vi "Write FPGA Outputs.vi"(0 "FPGA Ref":T1, 1 "Tank CMDs":T2, 2 "App Config":T3={"Location"="", "Profiles Path"=path "", "Current Profile"="", "CA Number"="", "Controller Type:"=enum."Kuhnke", "Stagger Time (ms)"=0, "Tank 1 Fuel"="", "Tank 2 Fuel"="", "Serial Numbers"={"Position 1 SN"="", "Position 2 SN"="", "Poaition 3 SN"="", "Position 4 SN"="", "Position 5 SN"="", "Position 6 SN"=""}, "Pumps Present"={"Pump 1"=FALSE, "Pump 2"=FALSE, "Pump 3"=FALSE, "Pump 4"=FALSE, "Pump 5"=FALSE, "Pump 6"=FALSE}, "VoltCtrlRef"="", "VoltageSelect"=FALSE, "Watlow Present"=FALSE, "Temp 1"=0, "Temp 2"=0, "Voltage Scale"={"V_FFm"=10.0, "V_FFb"=0.0}, "Pressure Scale"={"Pres_FFm"=0.0, "Pres_FFb"=0.0}, "Temp Tolerance"=0.0, "Target Voltage"=0.0, "Target Pressure"=0.0, "Data Log Init"={"Data Path"=path "", "Data Log Rate (S/s)"=0, "AKLH Rate (Hours/S)"=0.0, "Sync Time Offset (min)"=0, "IP Last 3"=0, "WebDAV IP"=""}, "Email Handler IP"="", "ADC Check"=FALSE, "3 Pump Tank"=FALSE, "Freq Flow?"=FALSE, "Profile Temp Control"=FALSE, "Read Controller Diag"=FALSE, "FFT Min Freq."=0, "FFT Max Freq."=0, "Speed by Current"=FALSE, "Watlow is F4T?"=FALSE, "Test Stop Time"=0.0, "Stop Time Enable"=TRUE, "Timers Include Off-Time"=FALSE, "Pump Timer Email"={"Enable"=FALSE, "Hour to Send"=0}, "Reset Step on Startup"=FALSE}, 3 "Power Relay":T7, 5 "Voltage Enable":bool, 6 "Run Profile":bool) -> (14 "FPGA Ref OUT":T1)   [LabVIEW 2019]
uses:
  Type Defs/App Config.ctl
  Type Defs/Controller Names.ctl
  Data Logger/Data Log Init.ctl
  Type Defs/Pump Timer Email.ctl
  Controls/Tank CMDs.ctl
  Controls/FPGA_Reference.ctl
  <vilib>/Utility/error.llb/Error Cluster From Error Code.vi
  <vilib>/rvi/errors/niLvFpgaAdjustHostInterfaceError.vi
  <vilib>/rvi/interface/nirviReadWriteControl/nirviReadWriteControl.xnode
  FPGA/bitfiles/TI sbRIO PWM (FPGA) v1.0.lvbitx
  NiFpgaLv.dll
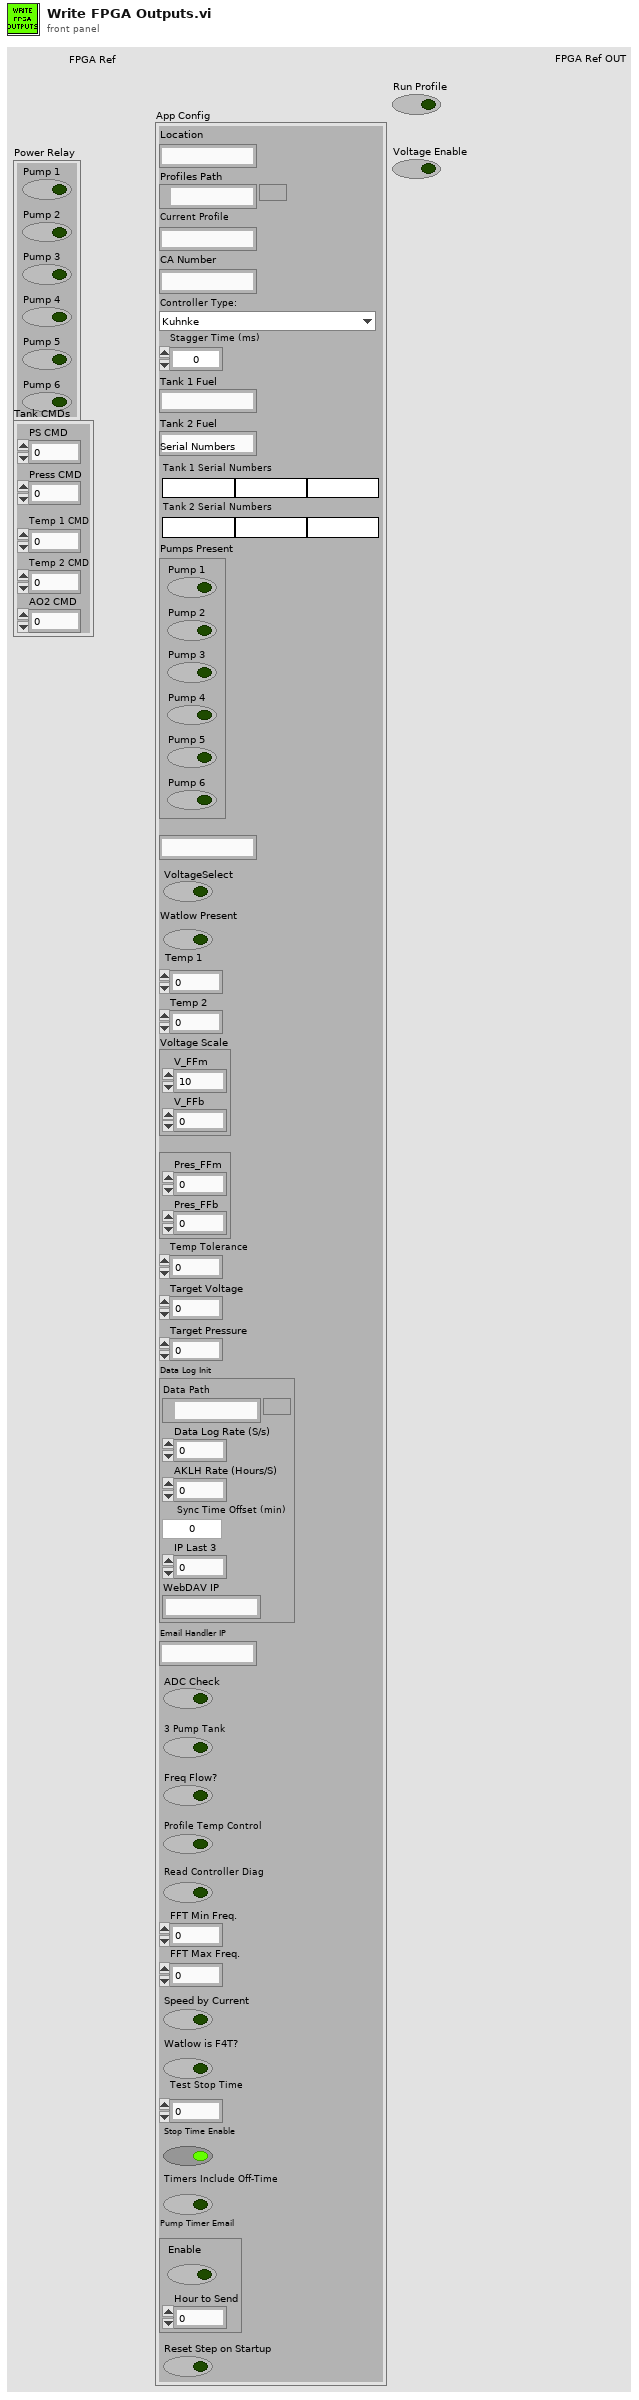
[diagram p1: front panel]
types:
  T1 = typedef "FPGA_Reference.ctl" = refnum<k20>
  T2 = typedef "Tank CMDs.ctl" = cluster{"PS CMD":dbl, "Press CMD":dbl, "Temp 1 CMD":dbl, "Temp 2 CMD":dbl, "AO2 CMD":dbl}
  T3 = typedef "App Config.ctl" = cluster{"Location":string, "Profiles Path":path, "Current Profile":string, "CA Number":string, "Controller Type:":T4, "Stagger Time (ms)":i32, "Tank 1 Fuel":string, "Tank 2 Fuel":string, "Serial Numbers":cluster{"Position 1 SN":string, "Position 2 SN":string, "Poaition 3 SN":string, "Position 4 SN":string, "Position 5 SN":string, "Position 6 SN":string}, "Pumps Present":cluster{"Pump 1":bool, "Pump 2":bool, "Pump 3":bool, "Pump 4":bool, "Pump 5":bool, "Pump 6":bool}, "VoltCtrlRef":string, "VoltageSelect":bool, "Watlow Present":bool, "Temp 1":i16, "Temp 2":i16, "Voltage Scale":cluster{"V_FFm":dbl, "V_FFb":dbl}, "Pressure Scale":cluster{"Pres_FFm":dbl, "Pres_FFb":dbl}, "Temp Tolerance":dbl, "Target Voltage":dbl, "Target Pressure":dbl, "Data Log Init":T5, "Email Handler IP":string, "ADC Check":bool, "3 Pump Tank":bool, "Freq Flow?":bool, "Profile Temp Control":bool, "Read Controller Diag":bool, "FFT Min Freq.":i32, "FFT Max Freq.":i32, "Speed by Current":bool, "Watlow is F4T?":bool, "Test Stop Time":dbl, "Stop Time Enable":bool, "Timers Include Off-Time":bool, "Pump Timer Email":T6, "Reset Step on Startup":bool}
  T4 = typedef "Controller Names.ctl" = enum16{"Kuhnke", "Helbako BLDC", "Conti", "Hella BLDC OL PWM", "Hella BLDC Turbine OL PWM", "Hella BLDC Pressure", "Helbako (old)", "TI PWM", "PSA", "Hella Gas", "Hella Diesel", "8 Comm", "10 Comm", "8 Comm Hella", "10 Comm Hella", "8 Comm Omron", "10 Comm Omron", "8 Comm Nissan", "10 Comm Nissan", "8 Comm Hella (for FCA)", "Mazda BLDC", "CMFB"}
  T5 = typedef "Data Log Init.ctl" = cluster{"Data Path":path, "Data Log Rate (S/s)":u32, "AKLH Rate (Hours/S)":dbl, "Sync Time Offset (min)":i32, "IP Last 3":i32, "WebDAV IP":string}
  T6 = typedef "Pump Timer Email.ctl" = cluster{"Enable":bool, "Hour to Send":u8}
  T7 = cluster{"Pump 1":bool, "Pump 2":bool, "Pump 3":bool, "Pump 4":bool, "Pump 5":bool, "Pump 6":bool}
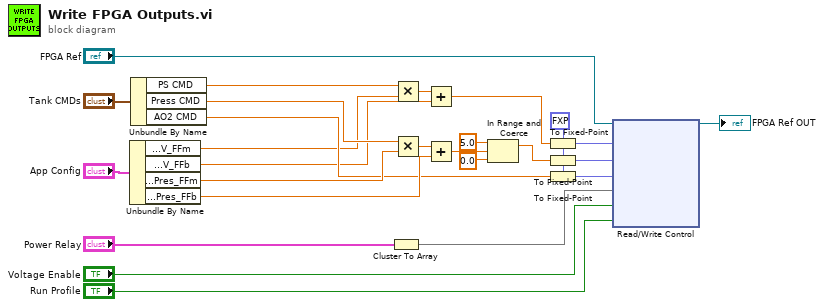
[diagram p0: block diagram]
diagram:
  w3 = fxp<+/-,20,5> 0.0 ("AO0")
  n1 = Unbundle By Name("App Config") -> ("Voltage Scale.V_FFm"=w5:dbl, "Voltage Scale.V_FFb"=w4:dbl, "Pressure Scale.Pres_FFm"=w16:dbl, "Pressure Scale.Pres_FFb"=w15:dbl)
  n2 = Unbundle By Name("Tank CMDs") -> ("PS CMD"=w6:dbl, "Press CMD"=w18:dbl, "AO2 CMD"=w10:dbl)
  n3 = Cluster To Array(cluster="Power Relay") -> (array=w9:bool[])
  n4 = Multiply(x=w6, y=w5) -> (x*y=w7:dbl)
  n5 = Multiply(x=w18, y=w16) -> (x*y=w25:dbl)
  n6 = Add(x=w7, y=w4) -> (x+y=w1:dbl)
  n7 = Add(x=w25, y=w15) -> (x+y=w26:dbl)
  n8 = In Range and Coerce(upper limit=5.0, x=w26, lower limit=0.0) -> (coerced(x)=w22:dbl)  [unwired: 1 out]
  n9 = To Fixed-Point(fixed-point type=w3, number=w1) -> (fixed-point=w2:fxp<+/-,20,5>)
  n10 = To Fixed-Point(fixed-point type=w3, number=w22) -> (fixed-point=w8:fxp<+/-,20,5>)
  n11 = To Fixed-Point(fixed-point type=w3, number=w10) -> (fixed-point=w11:fxp<+/-,20,5>)
  n12 = xnode "Read/Write Control"("FPGA VI Reference In"="FPGA Ref", "PS Cmd"=w2, "Pressure Cmd"=w8, "AO2"=w11, "Power Relays"=w9, "DIO18"="Voltage Enable", "DIO22"="Run Profile") -> ("FPGA VI Reference Out"=→"FPGA Ref OUT":T1)  [unwired: 1 in, 1 out]
